vi "Mean_and_Variance_Stats.vi"(4 "Block No":i32=1, 5 "Shift in":dbl[](array[numeric]) format="%.2f", 8 "U":dbl[](array[numeric]) format="%.2f") -> (0 "Shift out":dbl[](array[numeric]) format="%.2f", 2 "u^2":dbl, 3 "U":dbl)   [LabVIEW 2011]
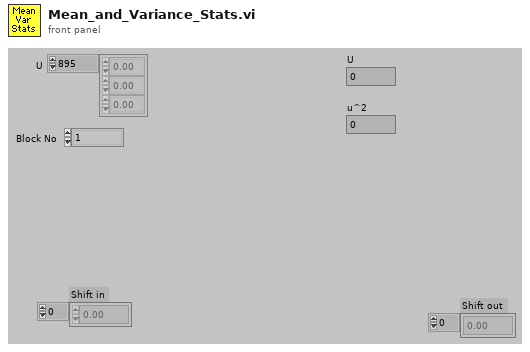
[diagram p1: front panel]
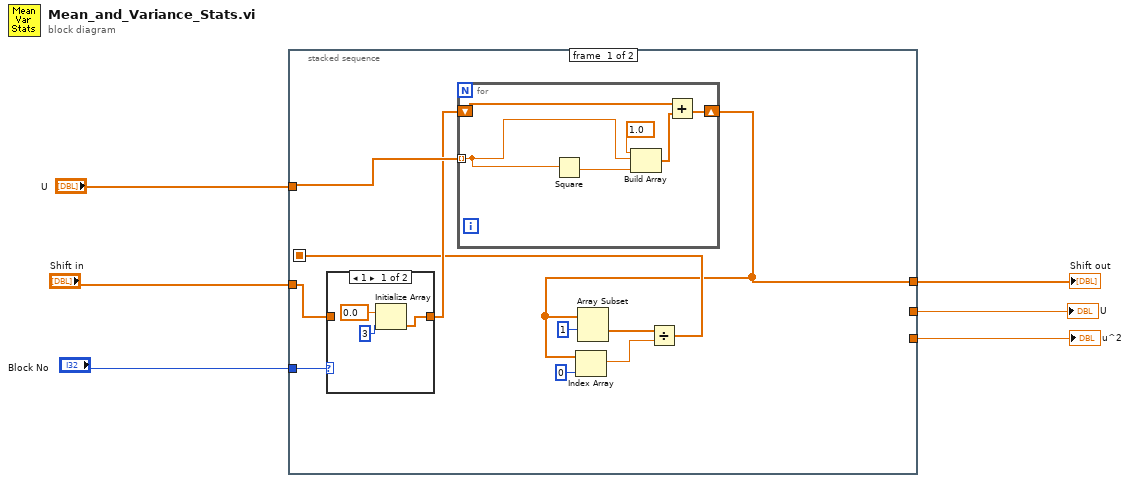
[diagram p0: block diagram]
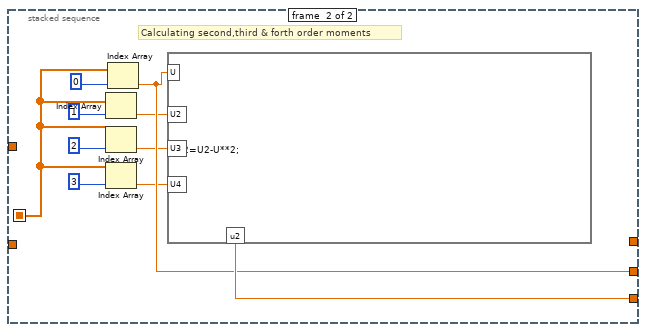
[diagram p3: hidden frame]
diagram:
  n1 = stacked-sequence {
    seq-local: [w8 _] -> [_ w34]
    tunnel: "U" -> [w16 _]
    tunnel: [w7 _] -> w5
    tunnel: "Shift in" -> [w10 _]
    tunnel: "Block No" -> [w11 _]
    tunnel: [_ w30] -> w2
    tunnel: [_ w31] -> w1
    frame #0 {
      n2 = case shown="1" w11 {
        tunnel: [w17 w20] -> w9
        tunnel: w10 -> [_ w20]
        frame 1 {
          n3 = Initialize Array(0.0 ("Element Data"), 3 ("Dimension Size")) -> (w17:dbl[])
        }
        frame 2, Default {
        }
      }
      n4 = for {
        shift-right: [w25] -> w7
        shift-left: w9 -> [w26]
        tunnel: w16 -> [w22] mode=indexing
        n5 = Square(x=w22) -> (x^2=w21:dbl)
        n6 = Build Array(1.0 ("Input Element"), w22, w21) -> (w24:dbl[])
        n7 = Add(x=w26, y=w24) -> (x+y=w25:dbl[])
      }
      n8 = Index Array(array=w7, index=0 ("Index")) -> (element=w12:dbl)
      n9 = Array Subset(array=w7, index=1 ("Array Index")) -> (w13:dbl[])  [unwired: 1 in]
      n10 = Divide(x=w13, y=w12) -> (x/y=w8:dbl[])
    }
    frame #1 {
      # "Calculating second,third & forth order moments"
      n11 = Index Array(array=w34, index=1) -> (element=w29:dbl)
      n12 = Index Array(array=w34, index=2) -> (element=w28:dbl)
      n13 = Index Array(array=w34, index=3) -> (element=w27:dbl)
      n14 = Index Array(array=w34, index=0) -> (element=w30:dbl)
      n15 = formula code="u2=U2-U**2;"("U"=w30, "U2"=w29, "U3"=w28, "U4"=w27) -> ("u2"=w31:dbl)
    }
  }
  "Shift out" <- w5
  "U" <- w2
  "u^2" <- w1
